vi "subvi.vi"(9 "NAO1":u32, 10 "Memory label":refnum<k21>, 11 "AO channel":refnum<k21>) -> ()   [LabVIEW 2016]
uses:
  <vilib>/rvi/Emulation/niFpgaGetClockAttributes.vi
  <vilib>/rvi/Emulation/niFpgaSctlEmulationGetInTimedLoop.vi
  <vilib>/rvi/Emulation/niFpgaEmulationReportErrorSimple.vi
  <vilib>/rvi/DataTransferAndStorage/Container/Common/niFpgaContainerExecOnDevCompGetState.vi
  <vilib>/rvi/Emulation/niFpgaEmulationIsFPGAContextNoSignature.vi
  <vilib>/rvi/DataTransferAndStorage/Container/Common/niFpgaContainerGetUniqueNameForEmu.vi
  <vilib>/rvi/Emulation/niFpgaProcessEmulError.vi
  <vilib>/rvi/errors/nirviReportUnexpectedCaseInternalError (U32).vi
  <vilib>/rvi/Memory/Memory_Emulation/niFpgaMemoryEmulationCacheClearOnFirstRun.vi
  <vilib>/rvi/Memory/Memory_Emulation/nirvimemoryEmulationManagerCache_MakeExclusive.vi
  <vilib>/rvi/Memory/Memory_Emulation/niFpgaMemoryEmulationValidateCache.vi
  <vilib>/rvi/Memory/Memory_Emulation/nirvimemoryEmulationManagerCache_InsertValue.vi
  <vilib>/Utility/error.llb/Clear Errors.vi
  <vilib>/rvi/Memory/Memory_Emulation/nirvimemoryEmulationManagerCache_ReleaseExclusive.vi
  <vilib>/rvi/Memory/Memory_Emulation/nirvimemoryEmulationManagerCache_GetValue.vi
  <vilib>/rvi/Memory/Memory_Emulation/nirvimemoryEmulationManagerCache_SetValue.vi
  <vilib>/rvi/Emulation/niFpgaSctlEmulationResourceMgr.vi
  <vilib>/rvi/eio/common/nirviEmuTemplateMethod_errors.vi
  <vilib>/rvi/Emulation/niFpgaCriticalErrorInLSC.vi
  <vilib>/rvi/DataTransferAndStorage/Container/XNode/niFpgaContainer.xnode
  <vilib>/rvi/Memory/Memory_Emulation/niFpgaMemoryEmulationRefIn.vi
  <vilib>/eio/EIONode/EIONode.xnode
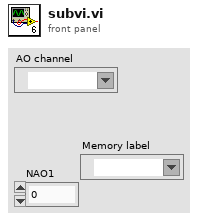
[diagram p1: front panel]
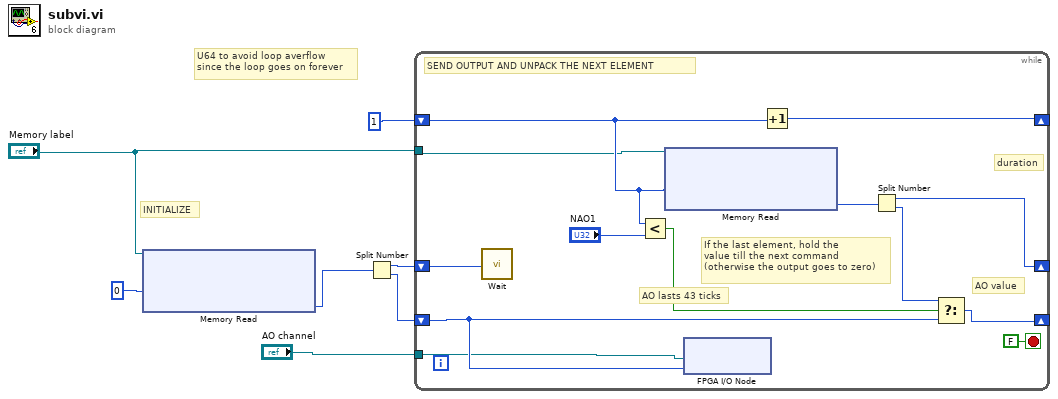
[diagram p0: block diagram]
diagram:
  # "INITIALIZE"
  # "U64 to avoid loop averflow\nsince the loop goes on forever"
  n1 = xnode ("Memory Read")("Memory In"="Memory label", "Address"=u32 0) -> ("Data"=w3:u32)  [unwired: 1 out]
  n2 = Split Number(x=w3) -> (hi(x)=w4:u16, lo(x)=w5:u16)
  n3 = while {
    shift-right: [w15] -> _
    shift-left: w4 -> [w20]
    shift-right: [w16] -> _
    shift-left: w5 -> [w13]
    shift-right: [w14] -> _
    shift-left: u64 1 -> [w11]
    tunnel: "AO channel" -> [w10]
    tunnel: "Memory label" -> [w9]
    stop <- FALSE stop-if-true
    # "duration"
    # "If the last element, hold the \nvalue till the next command\n(otherwise the output goes to zero)"
    # "AO lasts 43 ticks"
    # "AO value"
    # "SEND OUTPUT AND UNPACK THE NEXT ELEMENT"
    n4 = call "Wait"("Count(Ticks)"=w20) -> ()  [unwired: 1 out]
    n5 = Less?(x=w11, y="NAO1") -> (x < y?=w19:bool)
    n6 = xnode ("Memory Read")("Memory In"=w9, "Address"=w11) -> ("Data"=w12:u32)  [unwired: 1 out]
    n7 = xnode "FPGA I/O Node"("I/O Item"=w13, "FPGA I/O In"=w10) -> ()  [unwired: 1 out]
    n8 = Increment(x=w11) -> (x+1=w14:u64)
    n9 = Split Number(x=w12) -> (hi(x)=w15:u16, lo(x)=w17:u16)
    n10 = Select(t=w17, s=w19, f=w13) -> (s? t:f=w16:u16)
  }
